vi "LSX Get Calib Back Speed.vi"(8 "error in (no error)":errorcluster, 10 "plSpeed":i32, 11 "lLSID":i32) -> (0 "error out":errorcluster, 2 "plSpeed out":i32, 3 "function return":i32)   [LabVIEW 2018, in "Tango.lvlib"]
doc: "TANGOAPI int TANGOCALL LSX_GetCalibBackSpeed (int lLSID, int *plSpeed);"
uses:
  <userlib>/Tango/Tango.lvlib
  <userlib>/Tango/Tango_DLL.dll
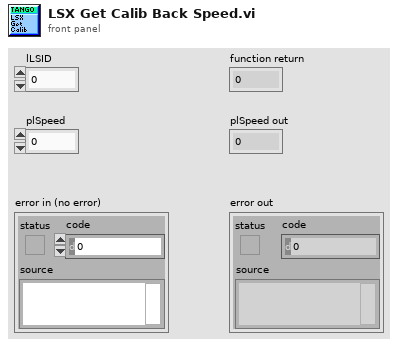
[diagram p1: front panel]
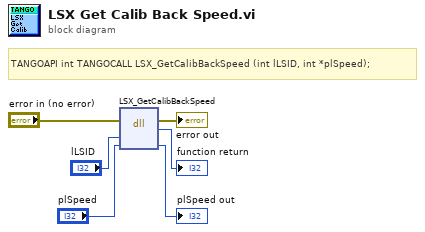
[diagram p0: block diagram]
diagram:
  # "TANGOAPI int TANGOCALL LSX_GetCalibBackSpeed (int lLSID, int *plSpeed);"
  n1 = dll-call lib="C:/Program Files (x86)/National Instruments/LabVIEW 2018/user.lib/Tango/Tango_DLL.*" fn="LSX_GetCalibBackSpeed"(error in="error in (no error)", "lLSID"="lLSID", "plSpeed"="plSpeed") -> (error out=→"error out":errorcluster, →"function return":i32, "plSpeed"=→"plSpeed out":i32)  [unwired: 3 in, 1 out]
